vi "Stall Force.vi"(6 "Skip Loading?":bool, 7 "Model Name":T1, 8 "Error In":errorcluster, 9 "Intialize?":bool=TRUE, 10 "Inputs":T2) -> (0 "error out":errorcluster, 1 "Completed":bool, 3 "Results":cluster{"Stall Force":dbl}, 4 "Status":cluster{"Status":string, "Elapsed Time":dbl})   [LabVIEW 2017]
uses:
  controls/All Inputs.ctl
  controls/SACB DI.ctl
  controls/Model Name.ctl
  controls/Stall Force.ctl
  controls/FGV DO.ctl
panel:
  in  "Wait for end":u32=500
  in  "Wait for Going Back":u32=100
  out "Numeric":dbl
  in  "Wait for Reading":u32=10
  out "Max Stall Force":dbl
  out "Average Stall Force":dbl
  out "Load Graph":dbl[](graph)
  in  "Tare Time":u32=500
  in  "Stall Force Read Time":u32=500
  in  "Delay (for Rest)":u32=500
  in  "Timeout (ms)":u32=15000
  # "Inputs"
  # "Variables"
  # "Outputs"
  # "Amount of time to take samples for stall reading"
  # "Amount of time to take samples for tare (initial reading)"
  # "Amount of time to wait before taking stall force reading"
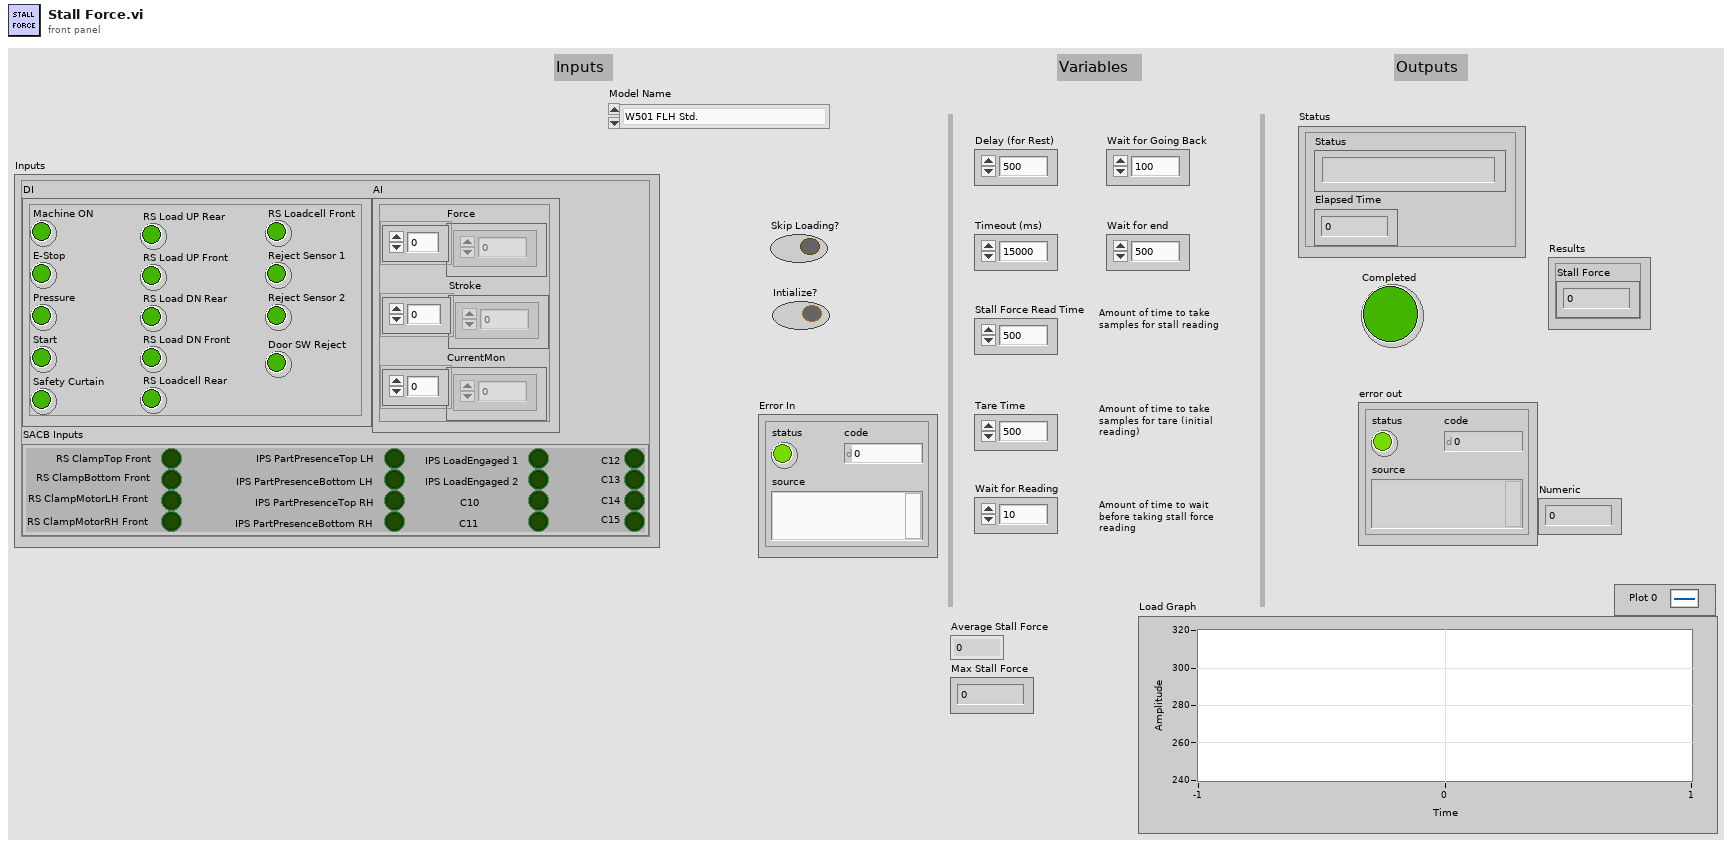
[diagram p1: front panel]
types:
  T1 = typedef "Model Name.ctl" = enum16{"W501 FLH Std.", "W501 FRH Std."}
  T2 = typedef "All Inputs.ctl" = cluster{"DI":cluster{"Machine ON":bool, "E-Stop":bool, "Pressure":bool, "Start":bool, "Safety Curtain":bool, "RS Load UP Rear":bool, "RS Load UP Front":bool, "RS Load DN Rear":bool, "RS Load DN Front":bool, "RS Loadcell Rear":bool, "RS Loadcell Front":bool, "Reject Sensor 1":bool, "Reject Sensor 2":bool, "Door SW Reject":bool}, "AI":cluster{"Force":dbl[], "Stroke":dbl[], "CurrentMon":dbl[]}, "SACB Inputs":T3}
  T3 = typedef "SACB DI.ctl" = cluster{"RS ClampTop Front":bool, "RS ClampBottom Front":bool, "RS ClampMotorLH Front":bool, "RS ClampMotorRH Front":bool, "IPS PartPresenceTop LH":bool, "IPS PartPresenceBottom LH":bool, "IPS PartPresenceTop RH":bool, "IPS PartPresenceBottom RH":bool, "IPS LoadEngaged 1":bool, "IPS LoadEngaged 2":bool, "C10":bool, "C11":bool, "C12":bool, "C13":bool, "C14":bool, "C15":bool}
  T4 = typedef "Stall Force.ctl" = enum16{"Initialize", "Wait for Tare", "Go Down", "Wait for Going Back", "Turn off Supply 1", "Load Cell CYL Front", "Go UP", "Wait for Reading", "Read Stall Force", "Load Cell CYL Rear", "Wait for End", "Turn Off Supply 2", "Wait for Rest", "Done", "Error"}
  T5 = typedef "FGV DO.ctl" = enum16{"Initialize", "Start Task", "Clamping", "Load CYL", "Contactors", "Loadcell CYL", "BSL", "Read DO", "Clear Tasks", "Clear Task"}
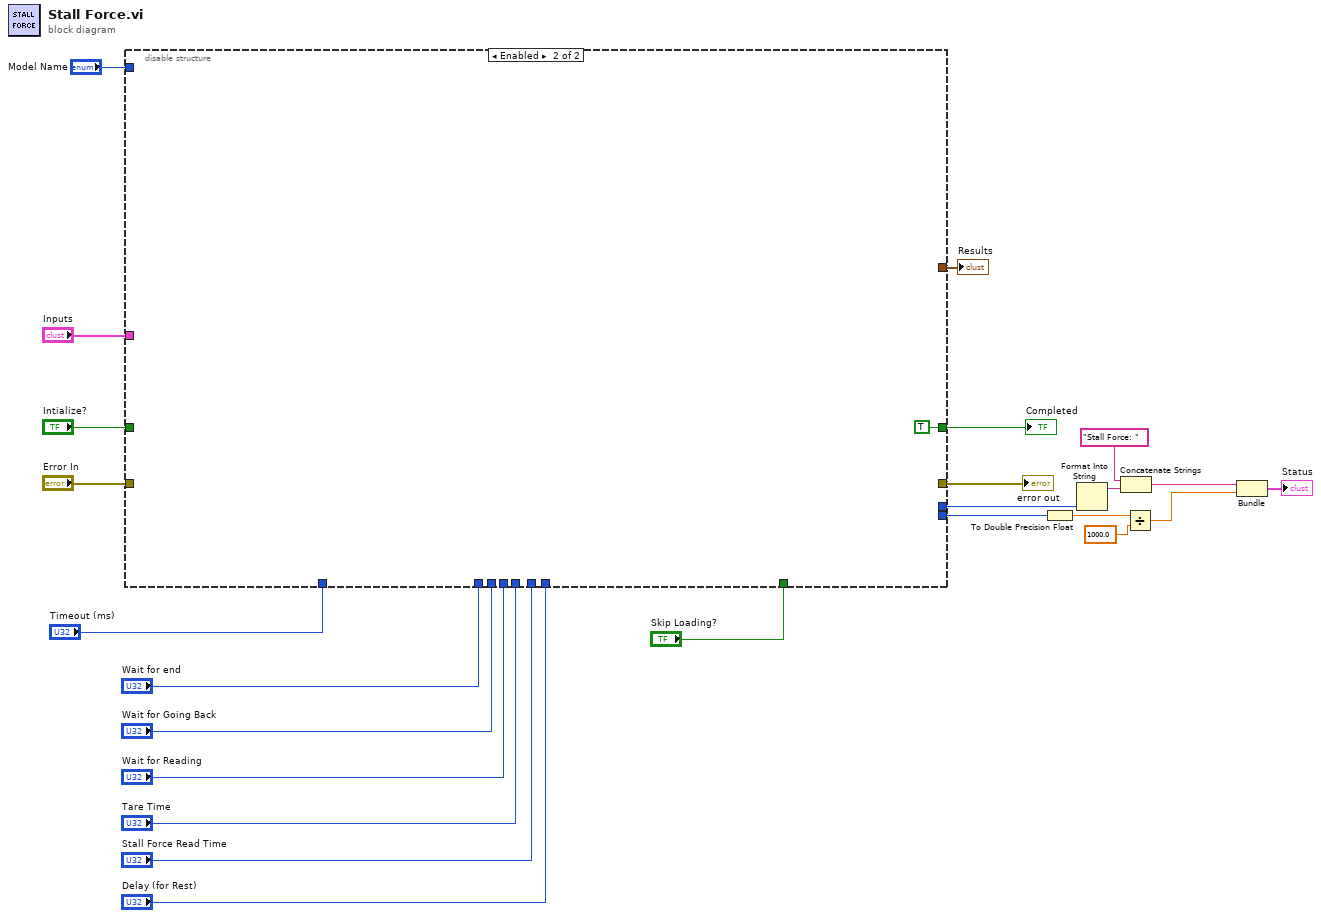
[diagram p0: block diagram]
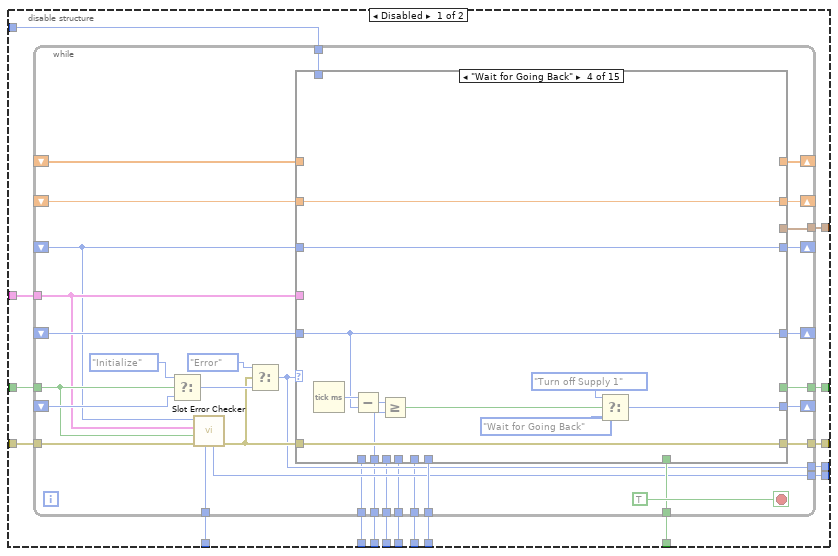
[diagram p2: hidden frame]
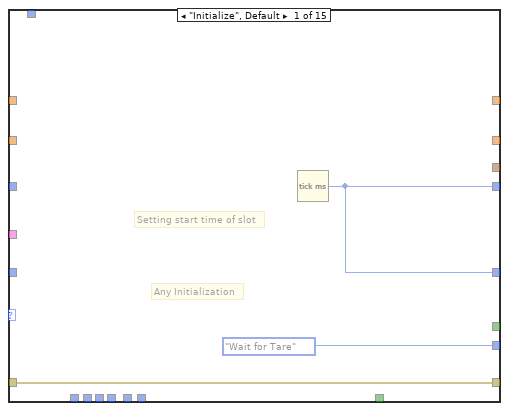
[diagram p3: hidden frame]
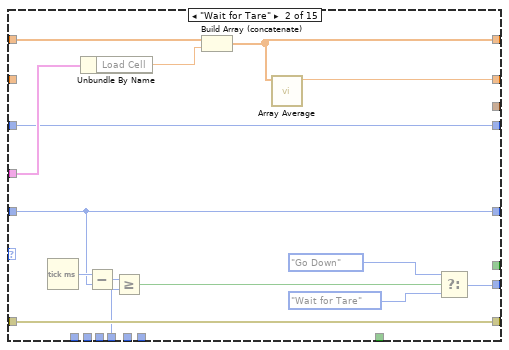
[diagram p4: hidden frame]
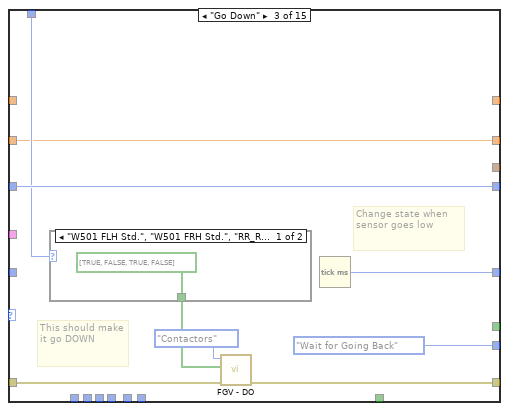
[diagram p5: hidden frame]
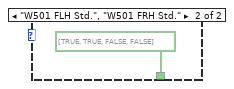
[diagram p6: hidden frame]
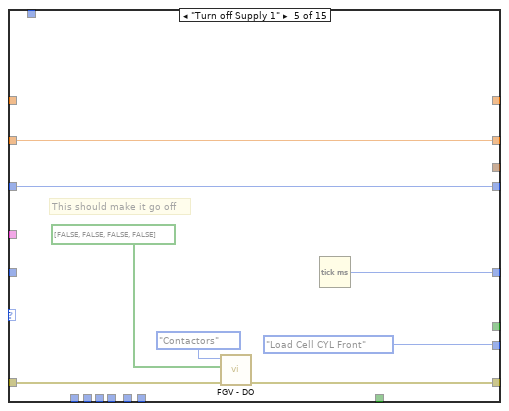
[diagram p7: hidden frame]
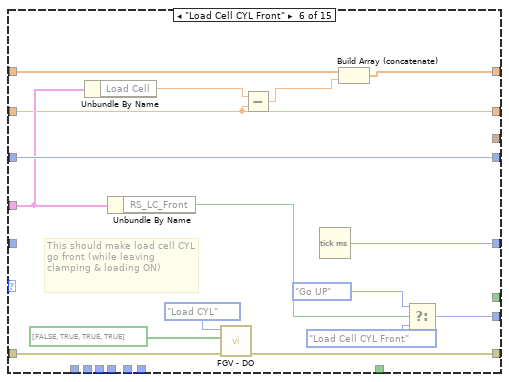
[diagram p8: hidden frame]
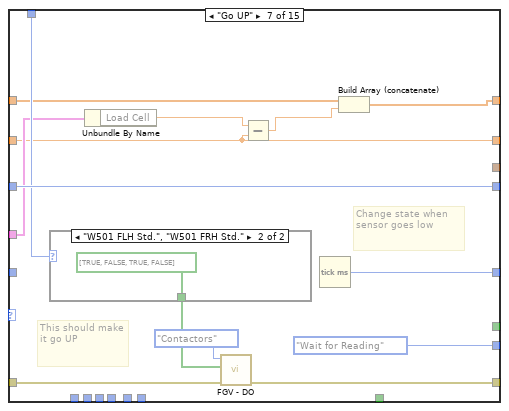
[diagram p9: hidden frame]
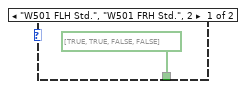
[diagram p10: hidden frame]
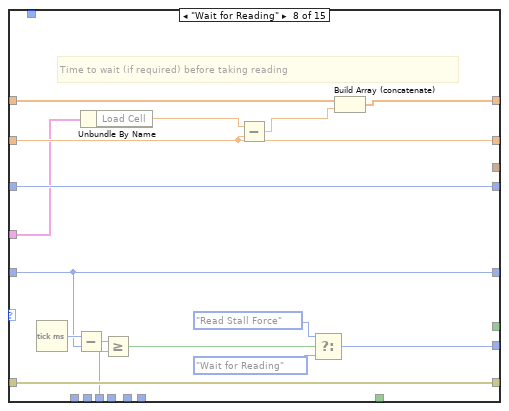
[diagram p11: hidden frame]
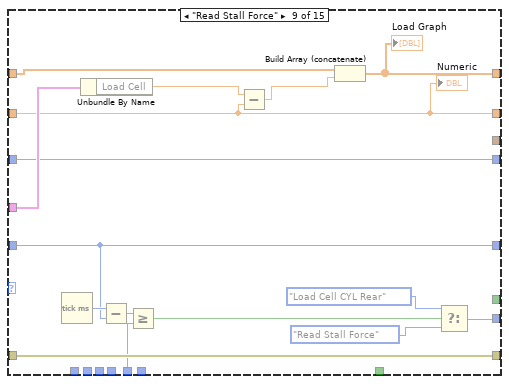
[diagram p12: hidden frame]
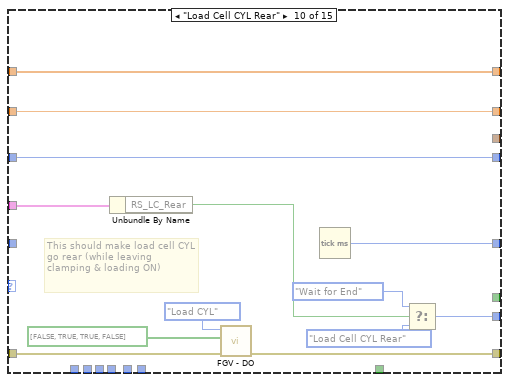
[diagram p13: hidden frame]
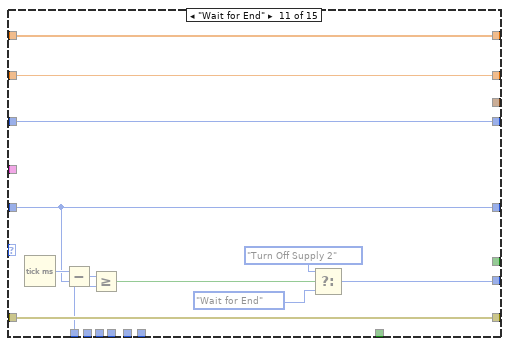
[diagram p14: hidden frame]
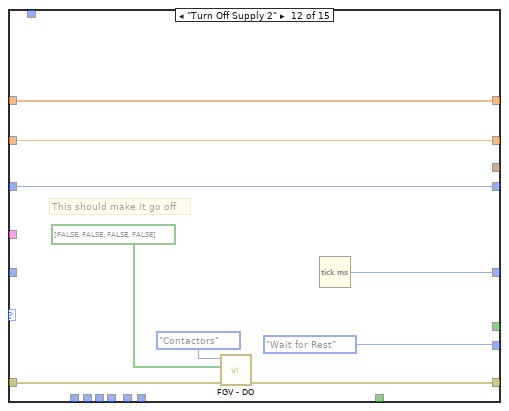
[diagram p15: hidden frame]
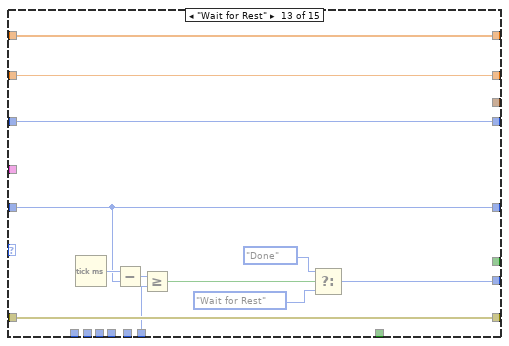
[diagram p16: hidden frame]
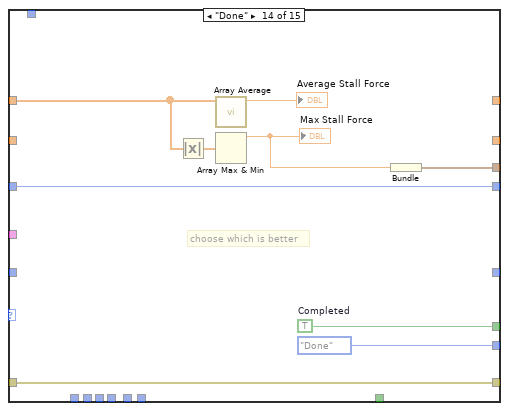
[diagram p17: hidden frame]
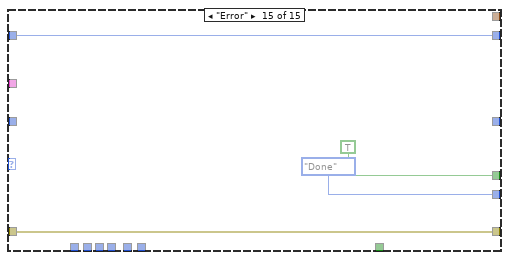
[diagram p18: hidden frame]
diagram:
  n1 = disable-structure shown="Enabled" {
    disable-tunnel: [w41 _] -> w24
    disable-tunnel: [w40 TRUE ("Completed")] -> w23
    disable-tunnel: "Inputs" -> [w39 _]
    disable-tunnel: "Error In" -> [w38 _]
    disable-tunnel: "Intialize?" -> [w37 _]
    disable-tunnel: "Delay (for Rest)" -> [w36 _]
    disable-tunnel: "Timeout (ms)" -> [w35 _]
    disable-tunnel: "Model Name" -> [w34 _]
    disable-tunnel: [w33 _] -> w16
    disable-tunnel: "Skip Loading?" -> [w32 _]
    disable-tunnel: [w31 _] -> w7
    disable-tunnel: [w30 _] -> w6
    disable-tunnel: "Stall Force Read Time" -> [w29 _]
    disable-tunnel: "Tare Time" -> [w28 _]
    disable-tunnel: "Wait for Reading" -> [w27 _]
    disable-tunnel: "Wait for end" -> [w26 _]
    disable-tunnel: "Wait for Going Back" -> [w25 _]
    frame Disabled {
      n2 = while {
        tunnel: w37 -> [w63]
        shift-right: [w70] -> _
        shift-left: _ -> [w72]
        shift-right: [w69] -> _
        shift-left: _ -> [w68]
        tunnel: w38 -> [w64]
        tunnel: [w67] -> w41
        tunnel: [w66] -> w40
        tunnel: w39 -> [w62]
        shift-right: [w65] -> _
        shift-left: _ -> [w61]
        tunnel: w36 -> [w57]
        tunnel: w35 -> [w56]
        tunnel: w34 -> [w55]
        shift-right: [w54] -> _
        shift-left: _ -> [w53]
        tunnel: [w52] -> w33
        tunnel: w32 -> [w51]
        shift-right: [w50] -> _
        shift-left: _ -> [w49]
        tunnel: [w48] -> w31
        tunnel: [w47] -> w30
        tunnel: w29 -> [w46]
        tunnel: w28 -> [w45]
        tunnel: w27 -> [w44]
        tunnel: w25 -> [w43]
        tunnel: w26 -> [w42]
        stop <- TRUE stop-if-true
        n3 = Select(t=Stall_Force."Initialize", s=w63, f=w72) -> (s? t:f=w60:T4)
        n4 = call "Slot Error Checker.vi"("Timeout (ms)"=w56, "error in (no error)"=w64, "Intialize?"=w63, "Inputs"=w62, "start time"=w61) -> ("error out"=w59:errorcluster, "Slot Time"=w48:u32)  [unwired: 5 in]
        n5 = Select(t=Stall_Force."Error", s=w59, f=w60) -> (s? t:f=w47:T4)
        n6 = case shown="\"Wait for Going Back\"" w47 {
          tunnel: [Stall_Force."Wait for Tare" w88 Stall_Force."Wait for Going Back" w110 Stall_Force."Load Cell CYL Front" w131 Stall_Force."Wait for Reading" w166 w182 w191 w207 Stall_Force."Wait for Rest" w228 Stall_Force."Done" Stall_Force."Done"] -> w70
          tunnel: [w74 w77 w94 w112 w116 w133 w145 w168 w175 w194 w209 w214 w230 _ _] -> w69
          tunnel: w68 -> [_ w77 _ w112 _ _ _ w168 w175 _ w209 _ w230 _ _]
          tunnel: w59 -> [w75 w91 w100 w108 w121 w137 w151 w164 w185 w198 w205 w219 w226 w239 w244]
          tunnel: [w75 w91 w99 w108 w120 w136 w150 w164 w185 w197 w205 w218 w226 w239 w244] -> w67
          tunnel: [_ _ _ _ _ _ _ _ _ _ _ _ _ w238 TRUE ("Completed")] -> w66
          tunnel: w62 -> [_ w87 _ _ _ w125 w139 w154 w181 w192 _ _ _ _ _]
          tunnel: [w74 w82 w96 w105 w115 w132 w147 w161 w177 w193 w202 w213 w223 w237 w241] -> w65
          tunnel: w61 -> [_ w82 w96 w105 w115 w132 w147 w161 w177 w193 w202 w213 w223 w237 w241]
          tunnel: w57 -> [_ _ _ _ _ _ _ _ _ _ _ _ w222 _ _]
          tunnel: w55 -> [_ _ w95 _ _ _ w146 _ _ _ _ _ _ _ _]
          tunnel: [_ w80 _ _ _ w123 w140 w156 w171 w186 w201 w212 w221 _ _] -> w54
          tunnel: w53 -> [_ w86 _ _ _ w122 w141 w157 w174 w186 w201 w212 w221 w235 _]
          tunnel: [_ _ _ _ _ _ _ _ _ _ _ _ _ w236 _] -> w52
          tunnel: w51 -> [_ _ _ _ _ _ _ _ _ _ _ _ _ _ _]
          tunnel: [_ w79 w92 w104 w114 w124 w138 w155 w170 w187 w200 w211 w220 _ _] -> w50
          tunnel: w49 -> [_ _ w92 w104 w114 w124 w138 w155 w170 w187 w200 w211 w220 _ _]
          tunnel: w46 -> [_ _ _ _ _ _ _ _ w178 _ _ _ _ _ _]
          tunnel: w45 -> [_ w78 _ _ _ _ _ _ _ _ _ _ _ _ _]
          tunnel: w44 -> [_ _ _ _ _ _ _ w160 _ _ _ _ _ _ _]
          tunnel: w43 -> [_ _ _ w103 _ _ _ _ _ _ _ _ _ _ _]
          tunnel: w42 -> [_ _ _ _ _ _ _ _ _ _ w199 _ _ _ _]
          frame "Initialize", Default {
            # "Setting start time of slot"
            # "Any Initialization"
            n7 = Tick Count (ms)() -> (millisecond timer value=w74:u32)
          }
          frame "Wait for Tare" {
            n8 = Tick Count (ms)() -> (millisecond timer value=w84:u32)
            n9 = Unbundle By Name(w87) -> ("Load Cell"=w85:dbl)
            n10 = Subtract(x=w84, y=w77) -> (x-y=w83:u32)
            n11 = Greater Or Equal?(x=w83, y=w78) -> (x >= y?=w81:bool)
            n12 = Build Array (concatenate)(w86, w85) -> (w80:dbl[])
            n13 = call "Array Average.vi"("data"=w80) -> ("Numeric"=w79:dbl)  [unwired: 10 in]
            n14 = Select(t=Stall_Force."Go Down", s=w81, f=Stall_Force."Wait for Tare") -> (s? t:f=w88:T4)
          }
          frame "Go Down" {
            # "Change state when sensor goes low"
            # "This should make it go DOWN"
            n15 = case shown="\"W501 FLH Std.\", \"W501 FRH Std.\", \"RR_RH_STD\"" w95 {
              tunnel: [bool[] [TRUE, FALSE, TRUE, FALSE] ("Digital Outs") bool[] [TRUE, TRUE, FALSE, FALSE] ("Digital Outs")] -> w97
              frame "W501 FLH Std.", "W501 FRH Std.", 2 {
              }
              frame "W501 FLH Std.", "W501 FRH Std." {
              }
            }
            n16 = call "FGV - DO.vi"("error in"=w100, "Digital Outs"=w97, "State"=FGV_DO."Contactors") -> ("error out"=w99:errorcluster)  [unwired: 7 in, 1 out]
            n17 = Tick Count (ms)() -> (millisecond timer value=w94:u32)
          }
          frame "Wait for Going Back" {
            n18 = Tick Count (ms)() -> (millisecond timer value=w113:u32)
            n19 = Subtract(x=w113, y=w112) -> (x-y=w111:u32)
            n20 = Greater Or Equal?(x=w111, y=w103) -> (x >= y?=w109:bool)
            n21 = Select(t=Stall_Force."Turn off Supply 1", s=w109, f=Stall_Force."Wait for Going Back") -> (s? t:f=w110:T4)
          }
          frame "Turn off Supply 1" {
            # "This should make it go off"
            n22 = call "FGV - DO.vi"("error in"=w121, "Digital Outs"=bool[] [FALSE, FALSE, FALSE, FALSE], "State"=FGV_DO."Contactors") -> ("error out"=w120:errorcluster)  [unwired: 7 in, 1 out]
            n23 = Tick Count (ms)() -> (millisecond timer value=w116:u32)
          }
          frame "Load Cell CYL Front" {
            # "This should make load cell CYL go front (while leaving clamping & loading ON)"
            n24 = Unbundle By Name(w125) -> ("Load Cell"=w127:dbl)
            n25 = Unbundle By Name(w125) -> ("RS_LC_Front"=w128:bool)
            n26 = call "FGV - DO.vi"("error in"=w137, "Digital Outs"=bool[] [FALSE, TRUE, TRUE, TRUE], "State"=FGV_DO."Load CYL") -> ("error out"=w136:errorcluster)  [unwired: 7 in, 1 out]
            n27 = Subtract(x=w127, y=w124) -> (x-y=w126:dbl)
            n28 = Tick Count (ms)() -> (millisecond timer value=w133:u32)
            n29 = Build Array (concatenate)(w122, w126) -> (w123:dbl[])
            n30 = Select(t=Stall_Force."Go UP", s=w128, f=Stall_Force."Load Cell CYL Front") -> (s? t:f=w131:T4)
          }
          frame "Go UP" {
            # "Change state when sensor goes low"
            # "This should make it go UP"
            n31 = case shown="\"FR_LH_STD\", \"RR_LH_STD\"" w146 {
              tunnel: [bool[] [TRUE, TRUE, FALSE, FALSE] ("Digital Outs") bool[] [TRUE, FALSE, TRUE, FALSE] ("Digital Outs")] -> w148
              frame "W501 FLH Std.", "W501 FRH Std.", 2 {
              }
              frame "W501 FLH Std.", "W501 FRH Std." {
              }
            }
            n32 = Unbundle By Name(w139) -> ("Load Cell"=w143:dbl)
            n33 = call "FGV - DO.vi"("error in"=w151, "Digital Outs"=w148, "State"=FGV_DO."Contactors") -> ("error out"=w150:errorcluster)  [unwired: 7 in, 1 out]
            n34 = Subtract(x=w143, y=w138) -> (x-y=w142:dbl)
            n35 = Tick Count (ms)() -> (millisecond timer value=w145:u32)
            n36 = Build Array (concatenate)(w141, w142) -> (w140:dbl[])
          }
          frame "Wait for Reading" {
            # "Time to wait (if required) before taking reading"
            n37 = Tick Count (ms)() -> (millisecond timer value=w169:u32)
            n38 = Subtract(x=w169, y=w168) -> (x-y=w167:u32)
            n39 = Unbundle By Name(w154) -> ("Load Cell"=w159:dbl)
            n40 = Greater Or Equal?(x=w167, y=w160) -> (x >= y?=w165:bool)
            n41 = Subtract(x=w159, y=w155) -> (x-y=w158:dbl)
            n42 = Select(t=Stall_Force."Read Stall Force", s=w165, f=Stall_Force."Wait for Reading") -> (s? t:f=w166:T4)
            n43 = Build Array (concatenate)(w157, w158) -> (w156:dbl[])
          }
          frame "Read Stall Force" {
            n44 = Tick Count (ms)() -> (millisecond timer value=w180:u32)
            n45 = Unbundle By Name(w181) -> ("Load Cell"=w173:dbl)
            n46 = Subtract(x=w180, y=w175) -> (x-y=w179:u32)
            n47 = Greater Or Equal?(x=w179, y=w178) -> (x >= y?=w176:bool)
            n48 = Subtract(x=w173, y=w170) -> (x-y=w172:dbl)
            n49 = Build Array (concatenate)(w174, w172) -> (w171:dbl[])
            "Load Graph" <- w171
            n50 = Select(t=Stall_Force."Load Cell CYL Rear", s=w176, f=Stall_Force."Read Stall Force") -> (s? t:f=w182:T4)
            "Numeric" <- w170
          }
          frame "Load Cell CYL Rear" {
            # "This should make load cell CYL go rear (while leaving clamping & loading ON)"
            n51 = Unbundle By Name(w192) -> ("RS_LC_Rear"=w188:bool)
            n52 = call "FGV - DO.vi"("error in"=w198, "Digital Outs"=bool[] [FALSE, TRUE, TRUE, FALSE], "State"=FGV_DO."Load CYL") -> ("error out"=w197:errorcluster)  [unwired: 7 in, 1 out]
            n53 = Tick Count (ms)() -> (millisecond timer value=w194:u32)
            n54 = Select(t=Stall_Force."Wait for End", s=w188, f=Stall_Force."Load Cell CYL Rear") -> (s? t:f=w191:T4)
          }
          frame "Wait for End" {
            n55 = Tick Count (ms)() -> (millisecond timer value=w210:u32)
            n56 = Subtract(x=w210, y=w209) -> (x-y=w208:u32)
            n57 = Greater Or Equal?(x=w208, y=w199) -> (x >= y?=w206:bool)
            n58 = Select(t=Stall_Force."Turn Off Supply 2", s=w206, f=Stall_Force."Wait for End") -> (s? t:f=w207:T4)
          }
          frame "Turn Off Supply 2" {
            # "This should make it go off"
            n59 = call "FGV - DO.vi"("error in"=w219, "Digital Outs"=bool[] [FALSE, FALSE, FALSE, FALSE], "State"=FGV_DO."Contactors") -> ("error out"=w218:errorcluster)  [unwired: 7 in, 1 out]
            n60 = Tick Count (ms)() -> (millisecond timer value=w214:u32)
          }
          frame "Wait for Rest" {
            n61 = Tick Count (ms)() -> (millisecond timer value=w231:u32)
            n62 = Subtract(x=w231, y=w230) -> (x-y=w229:u32)
            n63 = Greater Or Equal?(x=w229, y=w222) -> (x >= y?=w227:bool)
            n64 = Select(t=Stall_Force."Done", s=w227, f=Stall_Force."Wait for Rest") -> (s? t:f=w228:T4)
          }
          frame "Done" {
            w238 = TRUE  # Completed
            # "choose which is better"
            n65 = Absolute Value(x=w235) -> (abs(x)=w234:dbl[])
            n66 = call "Array Average.vi"("data"=w235) -> ("Numeric"=→"Average Stall Force":dbl)  [unwired: 10 in]
            n67 = Array Max & Min(array=w234) -> (max value=w233:dbl)  [unwired: 3 out]
            "Max Stall Force" <- w233
            n68 = Bundle(w233) -> (w236:cluster{dbl})  [unwired: 1 in]
          }
          frame "Error" {
          }
        }
      }
    }
    frame Enabled {
    }
  }
  "error out" <- w24
  "Completed" <- w23
  "Results" <- w16
  n69 = To Double Precision Float(number=w7) -> (double precision float=w12:dbl)
  n70 = Format Into String(w6) -> (resulting string=w14:string)  [unwired: 3 in, 1 out]
  n71 = Concatenate Strings("Stall Force: ", w14) -> (w10:string)
  n72 = Divide(x=w12, y=1000.0) -> (x/y=w9:dbl)
  n73 = Bundle(w10, w9) -> (→"Status":cluster{string, dbl})  [unwired: 1 in]
